vi "RankDiagrams.vi"(6 "error in":errorcluster, 9 "VI Interpreter in":refnum<class "VI Interpreter.lvclass">) -> (0 "error out":errorcluster, 3 "VI Interpreter out":refnum<class "VI Interpreter.lvclass">, 4 "Rank":cluster{"nodes":i32[]}[](array[cluster]))   [LabVIEW 2014, in "VI Interpreter.lvclass"]
uses:
  VI Interpreter.lvclass
  <vilib>/Utility/traverseref.llb/TRef TravTarget.ctl
  VI_AST/VI_AST.lvclass
  VI Interpreter.lvclass/VI Interpreter.ctl
  VI_AST/VI_AST.lvclass/VI_AST.ctl
  <vilib>/Utility/traverseref.llb/VI Scripting - Traverse.lvlib
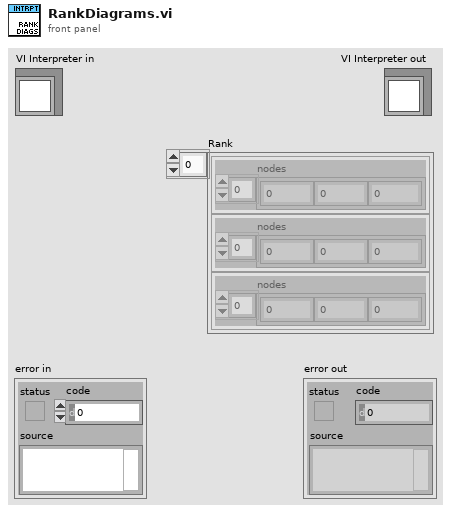
[diagram p1: front panel]
types:
  T1 = typedef "TRef TravTarget.ctl" = enum16{"FP", "BD", "Other"}
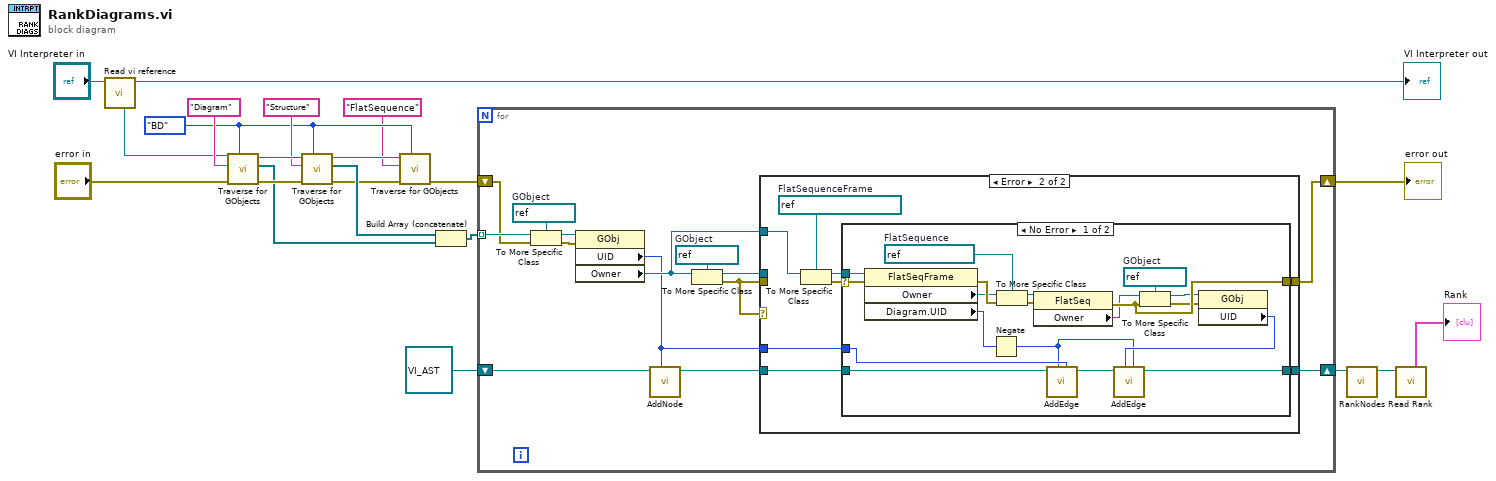
[diagram p0: block diagram]
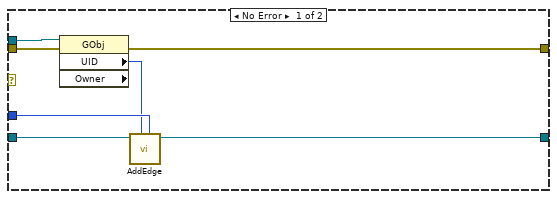
[diagram p2: hidden frame]
diagram:
  w11 = TRef_TravTarget."BD" ("Traverse Target")
  n1 = call "Read vi reference.vi"("VI Interpreter in"="VI Interpreter in") -> ("VI Interpreter out"=→"VI Interpreter out":refnum<class "VI Interpreter.lvclass">, "vi reference"=w8:refnum<vi>)  [unwired: 7 in]
  n2 = call <vilib>:"Traverse for GObjects.vi"("Traverse Target"=w11, "error in (no error)"="error in", "Class Name"="Diagram", "VI Refnum"=w8) -> ("error out"=w17:errorcluster, "References"=w15:refnum<vi>[], "dup VI Refnum"=w18:refnum<vi>)  [unwired: 4 in, 1 out]
  n3 = call <vilib>:"Traverse for GObjects.vi"("Traverse Target"=w11, "error in (no error)"=w17, "Class Name"="Structure", "VI Refnum"=w18) -> ("error out"=w10:errorcluster, "References"=w14:refnum<vi>[], "dup VI Refnum"=w12:refnum<vi>)  [unwired: 4 in, 1 out]
  n4 = call <vilib>:"Traverse for GObjects.vi"("Traverse Target"=w11, "error in (no error)"=w10, "Class Name"="FlatSequence", "VI Refnum"=w12) -> ("error out"=w4:errorcluster)  [unwired: 4 in, 3 out]
  n5 = Build Array (concatenate)(w14, w15) -> (w13:refnum<vi>[])
  n6 = for {
    tunnel: w13 -> [w35] mode=indexing
    shift-right: [w29] -> w6
    shift-left: refnum<class "VI_AST.lvclass"> refnum ("VI_AST in") -> [w24]
    shift-right: [w25] -> w3
    shift-left: w4 -> [w26]
    w31 = refnum<vi> refnum  # GObject
    w34 = refnum<vi> refnum  # GObject
    n7 = To More Specific Class(target class=w34, reference=w35, error in=w26) -> (specific class reference=w33:refnum<vi>, error out=w32:errorcluster)
    n8 = property class="GObj"(reference=w33, error in=w32) -> ("UID"=w22:i32, "Owner"=w27:refnum<vi>)  [unwired: 2 out]
    n9 = call "AddNode.vi"("UID"=w22, "VI_AST in"=w24) -> ("VI_AST out"=w23:refnum<class "VI_AST.lvclass">)  [unwired: 6 in, 1 out]
    n10 = To More Specific Class(target class=w31, reference=w27) -> (specific class reference=w30:refnum<vi>, error out=w28:errorcluster)  [unwired: 1 in]
    n11 = case shown="Error" w28 {
      tunnel: w28 -> [w42 _]
      tunnel: w30 -> [w41 _]
      tunnel: w23 -> [w37 w47]
      tunnel: w22 -> [w40 w44]
      tunnel: [w38 w45] -> w29
      tunnel: w27 -> [_ w50]
      tunnel: [w36 w43] -> w25
      frame No Error {
        n12 = property class="GObj" props=["UID", "Owner"](reference=w41, error in=w42) -> (error out=w36:errorcluster, "UID"=w39:i32)  [unwired: 2 out]
        n13 = call "AddEdge.vi"("sink"=w40, "source"=w39, "VI_AST in"=w37) -> ("VI_AST out"=w38:refnum<class "VI_AST.lvclass">)  [unwired: 6 in]
      }
      frame Error {
        w49 = refnum<vi> refnum  # FlatSequenceFrame
        n14 = To More Specific Class(target class=w49, reference=w50) -> (specific class reference=w46:refnum<vi>, error out=w48:errorcluster)  [unwired: 1 in]
        n15 = case shown="No Error" w48 {
          selector: w48 -> [w69 _]
          tunnel: w47 -> [w55 w70]
          tunnel: w46 -> [w68 _]
          tunnel: [w62 w70] -> w45
          tunnel: w44 -> [w53 _]
          tunnel: [w59 _] -> w43
          frame No Error {
            w60 = refnum<vi> refnum  # GObject
            w65 = refnum<vi> refnum  # FlatSequence
            n16 = property class="FlatSeqFrame"(reference=w68, error in=w69) -> (error out=w67:errorcluster, "Owner"=w66:refnum<vi>, "Diagram.UID"=w61:i32)  [unwired: 1 out]
            n17 = Negate(x=w61) -> (-x=w51:i32)
            n18 = To More Specific Class(target class=w65, reference=w66, error in=w67) -> (specific class reference=w64:refnum<vi>, error out=w63:errorcluster)
            n19 = property class="FlatSeq"(reference=w64, error in=w63) -> (error out=w59:errorcluster, "Owner"=w56:refnum<vi>)  [unwired: 1 out]
            n20 = call "AddEdge.vi"("sink"=w53, "source"=w51, "VI_AST in"=w55) -> ("VI_AST out"=w54:refnum<class "VI_AST.lvclass">)  [unwired: 6 in]
            n21 = To More Specific Class(target class=w60, reference=w56, error in=w59) -> (specific class reference=w58:refnum<vi>, error out=w57:errorcluster)
            n22 = property class="GObj"(reference=w58, error in=w57) -> ("UID"=w52:i32)  [unwired: 2 out]
            n23 = call "AddEdge.vi"("sink"=w51, "source"=w52, "VI_AST in"=w54) -> ("VI_AST out"=w62:refnum<class "VI_AST.lvclass">)  [unwired: 6 in]
          }
          frame Error {
          }
        }
      }
    }
  }
  "error out" <- w3
  n24 = call "RankNodes.vi"("VI_AST in"=w6) -> ("VI_AST out"=w2:refnum<class "VI_AST.lvclass">)  [unwired: 8 in]
  n25 = call "Read Rank.vi"("VI_AST in"=w2) -> ("Rank"=→"Rank":cluster{"nodes":i32[]}[])  [unwired: 7 in, 1 out]
